vi "Xctrl interface-Write X-Control data.vi"(7 "Reset graph X-axis scaling (F)":bool, 8 "error in (no error)":errorcluster, 9 "Data reference":refnum<data-value>) -> (0 "error out":errorcluster, 2 "Properties of selected ROI":cluster{"Type":T1, "Points per cycle":u16})   [LabVIEW 2013]
uses:
  Interface typedefs/Interface-ROI type enum.ctl
  Interface typedefs/Interface-Data array.ctl
  Interface typedefs/Interface-Data format definition.ctl
  Typedefs/Xctl-XY data type definition.ctl
  Typedefs/Xctrl-ROI type enum.ctl
  Interface typedefs/Interface-Data cluster.ctl
  XGrapher.xctl
  Global variables/gl_Functional Imaging-Global variables.vi
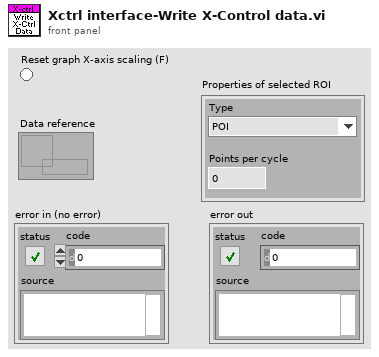
[diagram p1: front panel]
types:
  T1 = typedef "Interface-ROI type enum.ctl" = enum16{"POI", "Mini-scan"}
  T2 = typedef "Interface-Data cluster.ctl" = cluster{"Data & info by ROI index":T3, "Index of selected plot":u16, "Points in each trial":i32, "POI Averaging":bool, "Reset graph X-axis scaling":bool, "Selected point index in MSCN (unity based)":u16}
  T3 = typedef "Interface-Data array.ctl" = T4[]
  T4 = typedef "Interface-Data format definition.ctl" = cluster{"Plot.Plot Name":string, "Data":T5, "Timeline data":T5, "Type":T6, "Points per cycle":u16, "ROI number":u16}
  T5 = typedef "XGrapher.xctl/Xctl-XY data type definition.ctl" = cluster{"X-Axis values":sgl[], "Y-Axis values (s)":i32[]}
  T6 = typedef "Xctrl-ROI type enum.ctl" = enum16{"POI", "Mini-scan", "Group"}
  T7 = typedef "Functional Imging UI Refs.ctl" = cluster{"Menu ref":refnum<k9>, "Image control":refnum<vi>, "VI ref":refnum<vi>, "XGrapher":refnum<vi>, "Smoothing":refnum<vi>, "POI Averaging":refnum<vi>, "Normalize":refnum<vi>, "POI data points in each trial":refnum<vi>, "Channel":refnum<vi>, "Experiment data folder path":refnum<vi>, "[ROI vis]":refnum<vi>, "[Groups] visbl":T8, "Group Name":refnum<vi>, "POI index":refnum<vi>, "Trial No.":refnum<vi>, "Intensity Zoom":refnum<vi>, "Trial Cursor Enabled":refnum<vi>, "Number of Trials (ind 1)":refnum<vi>, "Number of Trials (ind 2)":refnum<vi>, "MiniScans Available":refnum<vi>, "POI Available":refnum<vi>, "Defer graph updates":refnum<vi>, "Waveform selector":refnum<vi>, "#of selected POI":refnum<vi>, "#of selected MiniScans":refnum<vi>, "#of selected groups":refnum<vi>, "Max Z-Projection":refnum<vi>, "Z-Plane Selector":refnum<vi>, "Index of miniscan point to visualise":refnum<vi>, "ROI vis. mode":refnum<vi>, "Total # of points":refnum<vi>, "Index of group clicked on":refnum<vi>, "Pane 1":refnum<vi>, "Pane 2":refnum<vi>, "Pane 3":refnum<vi>, "Pane 4":refnum<vi>, "Pane 5":refnum<vi>, "Pane 6":refnum<vi>, "Deselect all ROI":refnum<vi>, "Deselect all groups":refnum<vi>}
  T8 = typedef "Groups array referecne.ctl" = refnum<vi>
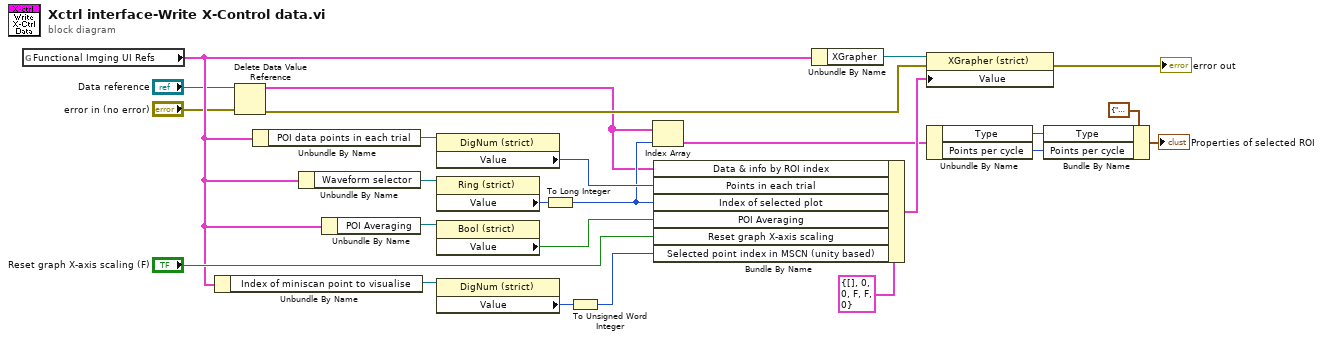
[diagram p0: block diagram]
diagram:
  n1 = global read "gl_Functional Imaging-Global variables.vi" "Functional Imging UI Refs"() -> (w11:T7)
  n2 = Unbundle By Name(w11) -> ("Index of miniscan point to visualise"=w19:refnum<vi>)
  n3 = Delete Data Value Reference(data value reference="Data reference", error in="error in (no error)") -> (data value=w1:T3, error out=w2:errorcluster)
  n4 = Unbundle By Name(w11) -> ("POI data points in each trial"=w24:refnum<vi>)
  n5 = Unbundle By Name(w11) -> ("Waveform selector"=w25:refnum<vi>)
  n6 = Unbundle By Name(w11) -> ("POI Averaging"=w22:refnum<vi>)
  n7 = property class="DigNum (strict)"(reference=w24) -> ("Value"=w23:i32)  [unwired: 1 in, 2 out]
  n8 = property class="Ring (strict)"(reference=w25) -> ("Value"=w16:u16)  [unwired: 1 in, 2 out]
  n9 = property class="Bool (strict)"(reference=w22) -> ("Value"=w21:bool)  [unwired: 1 in, 2 out]
  n10 = property class="DigNum (strict)"(reference=w19) -> ("Value"=w18:i32)  [unwired: 1 in, 2 out]
  n11 = To Long Integer(number=w16) -> (32bit integer=w15:i32)
  n12 = To Unsigned Word Integer(number=w18) -> (unsigned 16bit integer=w17:u16)
  n13 = Index Array(array=w1, index=w15) -> (element=w8:T4)
  n14 = Bundle By Name(cluster=T2 {"Data & info by ROI index"=[], "Index of selected plot"=0, "Points in each trial"=0, "POI Averaging"=FALSE, "Reset graph X-axis scaling"=FALSE, "Selected point index in MSCN (unity based)"=0} ("Value"), "Data & info by ROI index"=w1, "Points in each trial"=w23, "Index of selected plot"=w15, "POI Averaging"=w21, "Reset graph X-axis scaling"="Reset graph X-axis scaling (F)", "Selected point index in MSCN (unity based)"=w17) -> (w14:T2)
  n15 = Unbundle By Name(w11) -> ("XGrapher"=w12:refnum<vi>)
  n16 = property class="XGrapher (strict)"(reference=w12, error in=w2, "Value"=w14) -> (error out=→"error out":errorcluster)  [unwired: 1 out]
  n17 = Unbundle By Name(w8) -> ("Type"=w7:T6, "Points per cycle"=w6:u16)
  n18 = Bundle By Name(cluster=cluster{"Type":T1, "Points per cycle":u16} {"Type"=enum."POI", "Points per cycle"=0} ("Properties of selected ROI"), "Type"=w7, "Points per cycle"=w6) -> (→"Properties of selected ROI":cluster{"Type":T1, "Points per cycle":u16})
